vi "GSTOP CheckSet.vi"(1 "index(-1 for All)":i32=-1, 5 "stop value":bool, 7 "error in (no error)":errorcluster) -> (6 "stop":bool, 8 "error out":errorcluster)   [LabVIEW 2017, in "GSTOP.lvlib"]
doc: "Checks a Boolean input (typically wired to a Stop button) and triggers stop when the condition is met.\n------\n检查布尔输入（通常连接 Stop 按钮），并在满足条件时触发停止。"
uses:
  GSTOP.lvlib
  _def_oper.ctl
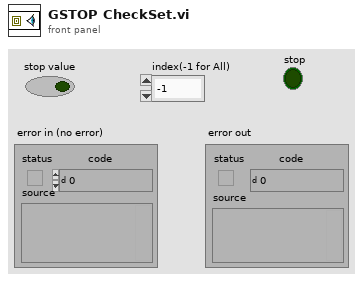
[diagram p1: front panel]
types:
  T1 = typedef "GSTOP.lvlib/_def_oper.ctl" = enum16{"init", "reset", "get", "set"}
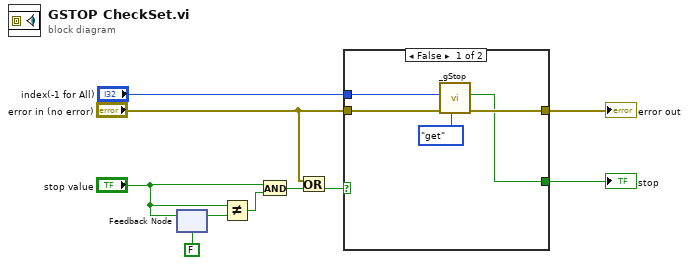
[diagram p0: block diagram]
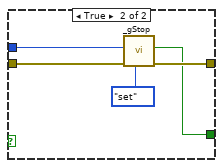
[diagram p2: hidden frame]
diagram:
  n1 = feedback-in #1("stop value") -> ()
  n2 = feedback #1(FALSE ("stop value")) -> (w9:bool)
  n3 = Not Equal?(x="stop value", y=w9) -> (x != y?=w8:bool)
  n4 = And(x="stop value", y=w8) -> (x .and. y?=w7:bool)
  n5 = Or(x="error in (no error)", y=w7) -> (x .or. y?=w3:bool)
  n6 = case shown="False" w3 {
    tunnel: "error in (no error)" -> [w14 w19]
    tunnel: [w13 w18] -> w5
    tunnel: [w12 w17] -> w4
    tunnel: "index(-1 for All)" -> [w11 w16]
    frame False {
      n7 = call "_gStop.vi"("op"=_def_oper."get", "error in (no error)"=w14, "index(-1 for All)"=w11) -> ("error out"=w13:errorcluster, "stop"=w12:bool)  [unwired: 7 in]
    }
    frame True {
      n8 = call "_gStop.vi"("op"=_def_oper."set", "error in (no error)"=w19, "index(-1 for All)"=w16) -> ("error out"=w18:errorcluster, "stop"=w17:bool)  [unwired: 7 in]
    }
  }
  "error out" <- w5
  "stop" <- w4
